vi "CANOpen.vi"(8 "error in (no error)":errorcluster caption="错误输入（无错误）", 10 "CAN Device In":T1={"Device Type"=20, "Device Index"=0, "CANInd"=0, "Baud(E_U)"=1835016} {"Baud(E_U)" items=["1000Kbps"=393219, "800Kbps"=393220, "500Kbps"=393223, "250Kbps"=1835016, "125Kbps"=1835025, "100Kbps"=1441827, "50Kbps"=1835052, "20Kbps"=1441971, "10Kbps"=1835232, "5Kbps"=1835457]; "Device Type" items=["PCI5121"=1, "PCI9810"=2, "USBCAN1"=3, "USBCAN2"=4, "PCI9820"=5, "PCI5110"=7, "PC104CAN"=11, "CANETUDP"=12, "PCI9840B"=14, "PC104C2"=15, "PCI9820I"=16, "CANETTCP"=17, "PCIE9221"=24, "PCI5010U"=19, "USBCAN_E_U"=20, "USBCAN_2E_U"=21, "PCI5020U"=22, "PCIE9120I"=27, "PCIE9110I"=28, "PCIE9140I"=29, "USBCAN-4E-U"=31, "USBCAN-8E-U"=34]}, 11 "ZLGCAN 输入":refnum<class "ZLGCAN.lvclass">) -> (0 "error out":errorcluster caption="错误输出", 3 "ZLGCAN 输出":refnum<class "ZLGCAN.lvclass">)   [LabVIEW 2020, in "ZLGCAN.lvclass"]
uses:
  ZLGCAN.lvclass
  ControlCAN/Device.ctl
  ZLGCAN.lvclass/ZLGCAN.ctl
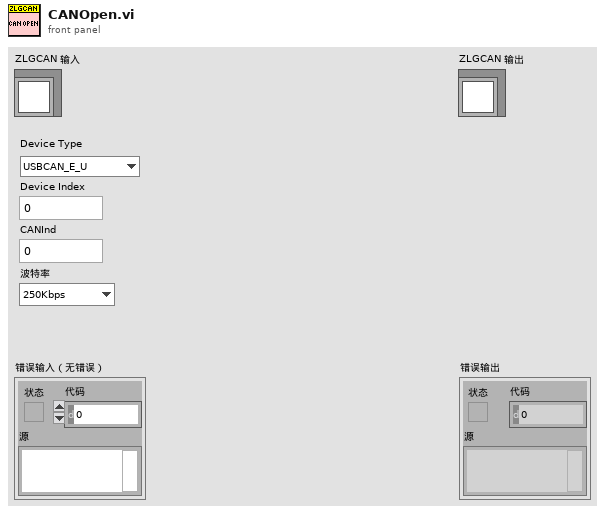
[diagram p1: front panel]
types:
  T1 = typedef "ZLGCAN.lvclass/Device.ctl" = cluster{"Device Type":u32, "Device Index":u32, "CANInd":u32, "Baud(E_U)":u32}
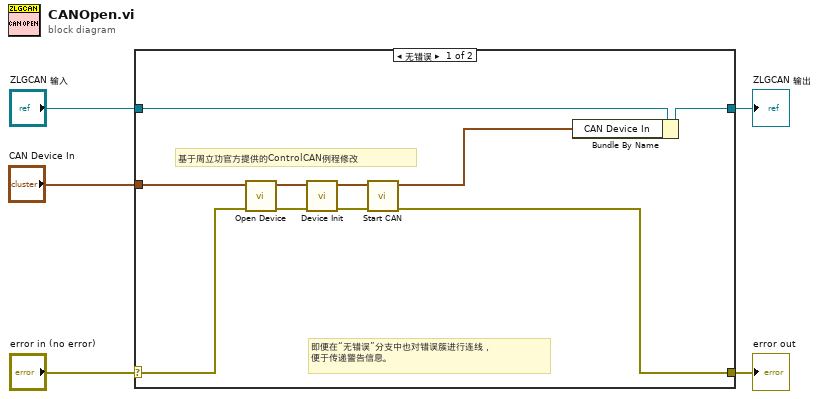
[diagram p0: block diagram]
diagram:
  n1 = case shown="无错误" "error in (no error)" {
    selector: "error in (no error)" -> [w12 w17]
    tunnel: [w7 w17] -> w4
    tunnel: [w8 w16] -> w2
    tunnel: "ZLGCAN 输入" -> [w15 w16]
    tunnel: "CAN Device In" -> [w10 _]
    frame No Error {
      # "基于周立功官方提供的ControlCAN例程修改"
      # "即便在“无错误”分支中也对错误簇进行连线，\n便于传递警告信息。"
      n2 = call "Open Device.vi"("错误输入（无错误）"=w12, "CAN Device In"=w10) -> ("错误输出"=w14:errorcluster, "CAN Device Out"=w11:T1)  [unwired: 7 in, 1 out]
      n3 = call "Device Init.vi"("错误输入（无错误）"=w14, "CAN Device In"=w11) -> ("错误输出"=w13:errorcluster, "CAN Device Out"=w9:T1)  [unwired: 8 in]
      n4 = call "Start CAN.vi"("错误输入（无错误）"=w13, "CAN Device In"=w9) -> ("错误输出"=w7:errorcluster, "CAN Device Out"=w6:T1)  [unwired: 7 in, 1 out]
      n5 = Bundle By Name(cluster=w15, "CAN Device In"=w6) -> (w8:refnum<class "ZLGCAN.lvclass">)
    }
    frame Error {
    }
  }
  "error out" <- w4
  "ZLGCAN 输出" <- w2
